vi "TimeChannel UTC (SubVI).vi"(11 "Waveform":waveform(dbl)) -> (1 "UTC Time SC DAQmx":u64[](array[numeric]), 2 "UTC Time FPGA":u64[](array[numeric]), 3 "Time waveform":waveform(dbl))   [LabVIEW 2019]
uses:
  <vilib>/Waveform/WDTOps.llb/WDT Number of Waveform Samples DBL.vi
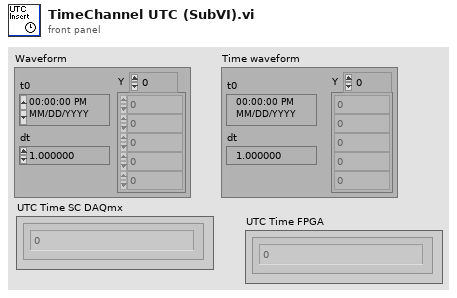
[diagram p1: front panel]
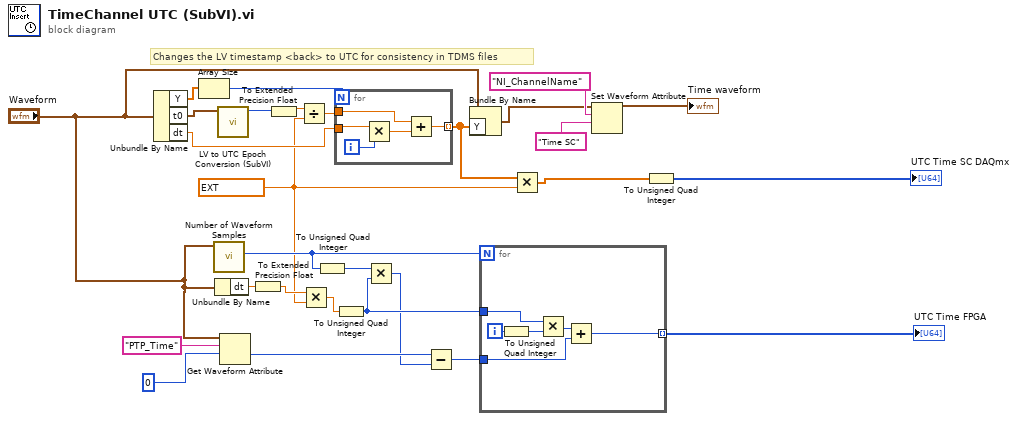
[diagram p0: block diagram]
diagram:
  w3 = ext 1000000000.0 ("y")
  # "Changes the LV timestamp <back> to UTC for consistency in TDMS files"
  n1 = Unbundle By Name("Waveform") -> ("Y"=w21:dbl[], "t0"=w2:timestamp, "dt"=w16:dbl)
  n2 = Array Size(array=w21) -> (size(s)=w22:i32)
  n3 = call-poly <vilib>:"Number of Waveform Samples.vi"("waveform in"="Waveform") -> ("number of samples"=w10:i32)  [unwired: 8 in, 2 out]
  n4 = Unbundle By Name("Waveform") -> ("dt"=w26:dbl)
  n5 = call "LV to UTC Epoch Conversion (SubVI).vi"("LabVIEW time"=w2) -> ("UTC time (ns)"=w1:u64)  [unwired: 10 in]
  n6 = Get Waveform Attribute(5:u64 0, 6:"PTP_Time" ("name"), 7:"Waveform") -> (1:w11:u64)  [unwired: 1 in, 3 out]
  n7 = To Extended Precision Float(1:w26) -> (0:w5:ext)
  n8 = To Extended Precision Float(1:w1) -> (0:w14:ext)
  n9 = Divide(x=w14, y=w3) -> (x/y=w15:ext)
  n10 = Multiply(x=w5, y=w3) -> (x*y=w27:ext)
  n11 = To Unsigned Quad Integer(1:w10) -> (0:w8:u64)
  n12 = for {
    N: w22 -> [_]
    tunnel: w16 -> [w32]
    tunnel: [w31] -> w13 mode=indexing
    tunnel: w15 -> [w30]
    i -> [w33]
    n13 = Multiply(x=w32, y=w33) -> (x*y=w29:dbl)
    n14 = Add(x=w30, y=w29) -> (x+y=w31:ext)
  }
  n15 = To Unsigned Quad Integer(1:w27) -> (0:w9:u64)
  n16 = Multiply(x=w8, y=w9) -> (x*y=w7:u64)
  n17 = Subtract(x=w11, y=w7) -> (x-y=w6:u64)
  n18 = Bundle By Name(cluster="Waveform", "Y"=w13) -> (w19:waveform(dbl))
  n19 = for {
    N: w10 -> [_]
    tunnel: w6 -> [w36]
    tunnel: w9 -> [w38]
    tunnel: [w35] -> w4 mode=indexing
    i -> [w39]
    n20 = To Unsigned Quad Integer(1:w39) -> (0:w34:u64)
    n21 = Multiply(x=w38, y=w34) -> (x*y=w37:u64)
    n22 = Add(x=w37, y=w36) -> (x+y=w35:u64)
  }
  "UTC Time FPGA" <- w4
  n23 = Multiply(x=w13, y=w3) -> (x*y=w28:ext[])
  n24 = Set Waveform Attribute(5:"Time SC", 6:"NI_ChannelName", 7:w19) -> (3:→"Time waveform":waveform(dbl))  [unwired: 1 in, 2 out]
  n25 = To Unsigned Quad Integer(1:w28) -> (0:→"UTC Time SC DAQmx":u64[])
